vi "DiffDriveTrainSim_ToughBoxMiniMotor.vi"(11 "ToughBoxMiniMotor":T2) -> (3 "DriveMotor":T1 {"Jr_KgM2" format="%13.5p"; "L_H" format="%13.5p"; "Kt_NMPerAmp" format="%13.5p"; "KvINV_RadPerSecPerVolt" format="%13.5p"; "R_Ohms" format="%13.5p"; "FreeSpeed_RadPerSec" format="%13.5p"; "FreeCurrent_Amps" format="%13.5p"; "StallCurrent_Amps" format="%13.5p"; "StallTorque_NM" format="%13.5p"; "nominalVoltage_Volts" format="%13.5p"})   [LabVIEW 2019, in "Trajectory_Library.lvlib"]
doc: "Convience function to allow user to select standard kit bot motor choices from an enum selector and return the motor data \n\nInput:\n - ToughBoxMiniMotor -- Enumerated motor selector\n\nOutput:\n - DriveMotor -- Selected motor data."
uses:
  Trajectory_Library.lvlib
  DIFF_DRIVE_ToughBoxMini_MotorChoice_ENUM.ctl
  DCMOTOR.CTL
  DCMotor_New.vi
  VI/Units_RotationsPerMinuteToRadiansPerSecond.vi
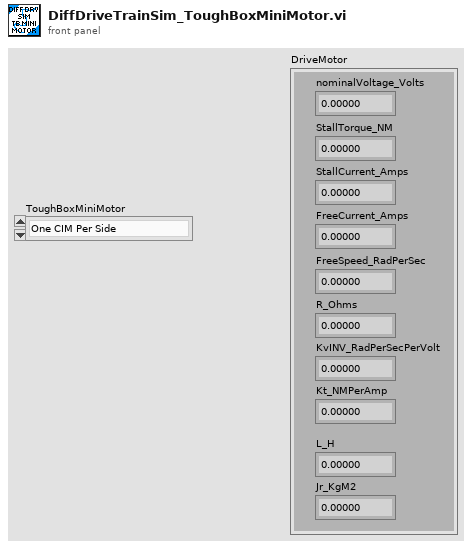
[diagram p1: front panel]
types:
  T1 = typedef "Trajectory_Library.lvlib/DCMOTOR.CTL" = cluster{"nominalVoltage_Volts":dbl, "StallTorque_NM":dbl, "StallCurrent_Amps":dbl, "FreeCurrent_Amps":dbl, "FreeSpeed_RadPerSec":dbl, "R_Ohms":dbl, "KvINV_RadPerSecPerVolt":dbl, "Kt_NMPerAmp":dbl, "L_H":dbl, "Jr_KgM2":dbl}
  T2 = typedef "Trajectory_Library.lvlib/DIFF_DRIVE_ToughBoxMini_MotorChoice_ENUM.ctl" = enum16{"One CIM Per Side", "Two CIM Per Side", "One MiniCIM Per Side", "Two Mini CIM Per Side", "Two Falcon Per Side", "Two NEO Per Side"}
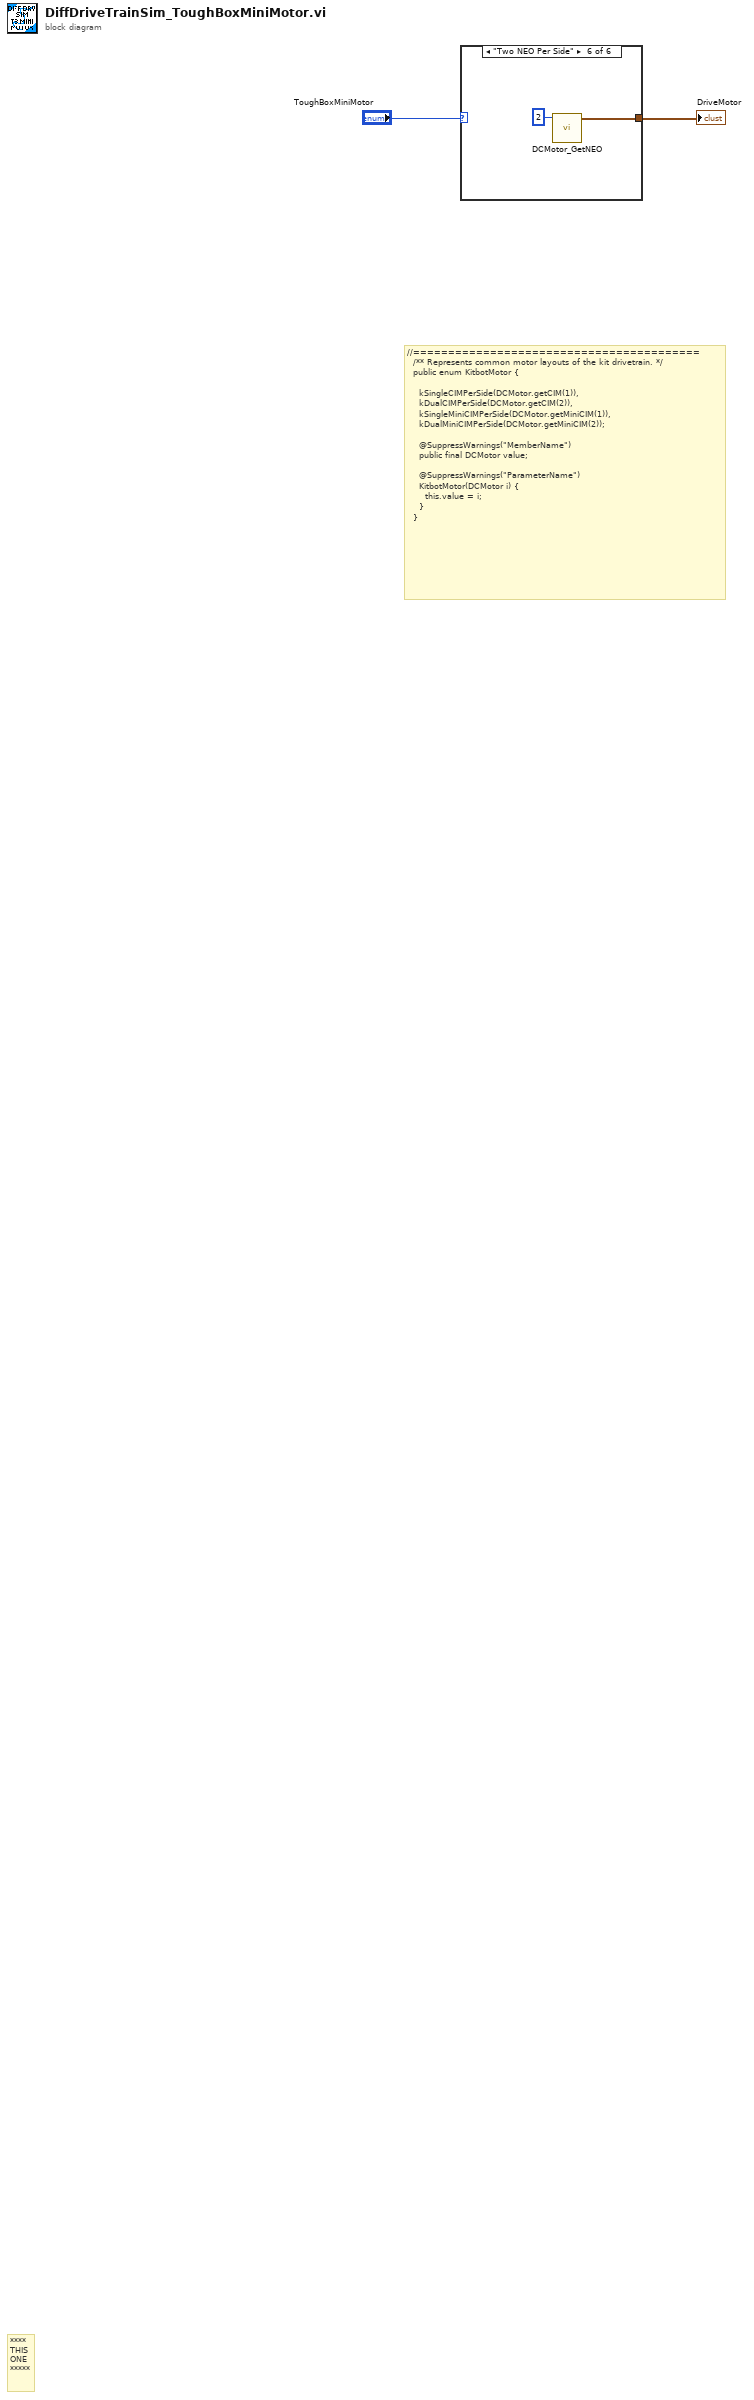
[diagram p0: block diagram]
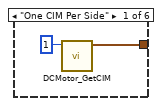
[diagram p2: hidden frame]
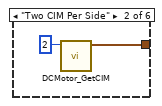
[diagram p3: hidden frame]
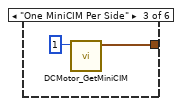
[diagram p4: hidden frame]
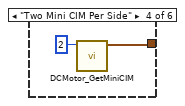
[diagram p5: hidden frame]
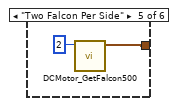
[diagram p6: hidden frame]
diagram:
  # "//=========================================\n  /** Represents common motor layouts of the kit drivetrain. */\n  public enum KitbotMotor {\n\n    kSingleCIMPerSide(DCMotor.getCIM(1)),\n    kDualCIMPerSide(DCMotor.getCIM(2)),\n    kSingleMiniCIMPerSide(DCMotor.getMiniCIM(1)),\n    kDualMiniCIMPerSide(DCMotor.getMiniCIM(2));\n\n    @SuppressWarnings(\"MemberName\")\n    public final DCMotor value;\n\n    @SuppressWarnings(\"ParameterName\")\n    KitbotMotor(DCMotor i) {\n      this.value = i;\n    }\n  }"
  # "****\nTHIS\nONE\n*****"
  n1 = case shown="\"Two NEO Per Side\"" "ToughBoxMiniMotor" {
    tunnel: [w3 w5 w7 w9 w12 w13] -> w1
    frame "One CIM Per Side" {
      n2 = call "DCMotor_GetCIM.vi"("Num Motors"=1) -> ("DCMOTOR"=w3:T1)  [unwired: 10 in]
    }
    frame "Two CIM Per Side" {
      n3 = call "DCMotor_GetCIM.vi"("Num Motors"=2) -> ("DCMOTOR"=w5:T1)  [unwired: 10 in]
    }
    frame "One MiniCIM Per Side" {
      n4 = call "DCMotor_GetMiniCIM.vi"("Num Motors"=1) -> ("DCMOTOR"=w7:T1)  [unwired: 10 in]
    }
    frame "Two Mini CIM Per Side" {
      n5 = call "DCMotor_GetMiniCIM.vi"("Num Motors"=2) -> ("DCMOTOR"=w9:T1)  [unwired: 10 in]
    }
    frame "Two Falcon Per Side" {
      n6 = call "DCMotor_GetFalcon500.vi"("Num Motors"=2) -> ("DCMOTOR"=w12:T1)  [unwired: 10 in]
    }
    frame "Two NEO Per Side" {
      n7 = call "DCMotor_GetNEO.vi"("Num Motors"=2) -> ("DCMOTOR"=w13:T1)  [unwired: 10 in]
    }
  }
  "DriveMotor" <- w1
